vi "filter.marvel_series.vi"(9 "filter char":string, 11 "marvel series map":map{i32, string}(c390)) -> (1 "series array":string[](array[string]), 3 "series map out":map{string, i32}(c390))   [LabVIEW 2024]
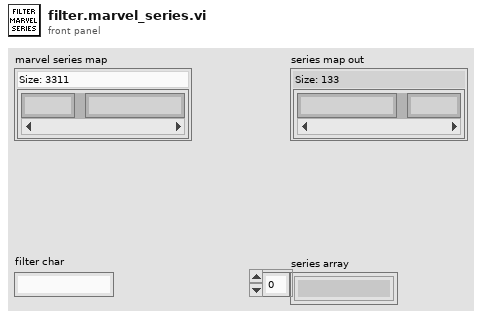
[diagram p1: front panel]
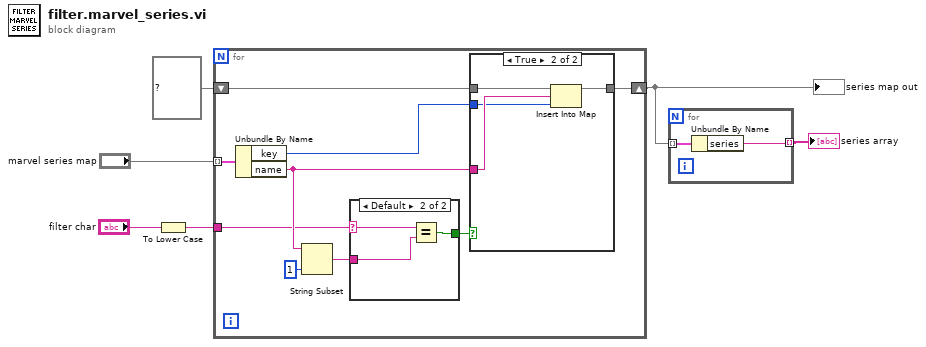
[diagram p0: block diagram]
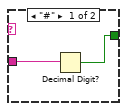
[diagram p2: hidden frame]
diagram:
  n1 = To Lower Case(string="filter char") -> (all lower case string=w6:string)
  n2 = for {
    tunnel: "marvel series map" -> [w15] mode=indexing
    tunnel: w6 -> [w12]
    shift-right: [w7] -> w3
    shift-left: map{string, i32} {} ("map") -> [w9]
    n3 = Unbundle By Name(w15) -> ("key"=w8:i32, "name"=w13:string)
    n4 = String Subset(string=w13, length (rest)=1 ("offset (0)")) -> (substring=w10:string)  [unwired: 1 in]
    n5 = case shown="Default" w12 {
      selector: w12 -> [_ w19]
      tunnel: [w16 w20] -> w14
      tunnel: w10 -> [w17 w18]
      frame "#" {
        n6 = Decimal Digit?(1:w17) -> (0:w16:bool)
      }
      frame Default {
        n7 = Equal?(x=w19, y=w18) -> (x = y?=w20:bool)
      }
    }
    n8 = case shown="True" w14 {
      tunnel: w13 -> [_ w25]
      tunnel: w9 -> [w21 w24]
      tunnel: w8 -> [_ w23]
      tunnel: [w21 w22] -> w7
      frame False {
      }
      frame True {
        n9 = Insert Into Map(map in=w24, key=w25, value=w23) -> (map out=w22:map{string, i32})  [unwired: 2 out]
      }
    }
  }
  "series map out" <- w3
  n10 = for {
    tunnel: w3 -> [w27] mode=indexing
    tunnel: [w26] -> w2 mode=indexing
    n11 = Unbundle By Name(w27) -> ("series"=w26:string)
  }
  "series array" <- w2
